vi "SPI API - SPI Simulation.vi"() -> ()   [LabVIEW 2014]
uses:
  Controls/Digital Data.ctl
  Controls/Timing Characteristics.ctl
panel:
  in  "SPI PHY Settings":T1={"Divide Value"=10, "Transfer Length (bits)"=24, "CS Asserted Polarity"=FALSE, "Clock Polarity (CPOL)"=FALSE, "Clock Phase (CPHA)"=FALSE, "Lengthen MISO Setup"=FALSE, "Direction Change Bit"=0, "MOSI Starts as Output"=FALSE, "Tristatable MOSI"=FALSE}
  in  "Chip Select":u8
  in  "Engine Rate (MHz)":i32=120
  out "Data To Slave":u64 format="%b"
  out "Timing Characteristics":T2 {"tCL (ns)" format="%#_4g"; "tCH (ns)" format="%#_4g"; "tCSS (ns)" format="%#_4g"; "tCSH (ns)" format="%#_4g"; "tCSW (ns)" format="%#_4g"; "Actual Sample Rate (Hz)" format="%_4p"; "SCLK Frequency (Hz)" format="%#.2p"}
  in  "Pause":bool
  in  "Sample Rate (Hz)":u32=100000 format="%.0p"
  out "Digital Data":digitalwaveform(graph)
  in  "Data To Slave":u64 format="%x"
  in  "Stop":bool
  # "Operating Instructions\n1. For this VI to work, the FPGA must be in Simulation Mode.\n2. Set the 'Engine Rate' control value to match your FPGA SPI Engine loop rate.\n3. Select a sample rate to control how often the SPI message is transmitted.\n4. Run the VI and observe the Timing Characterstics to the right."
  # "Typical Timing Diagram"
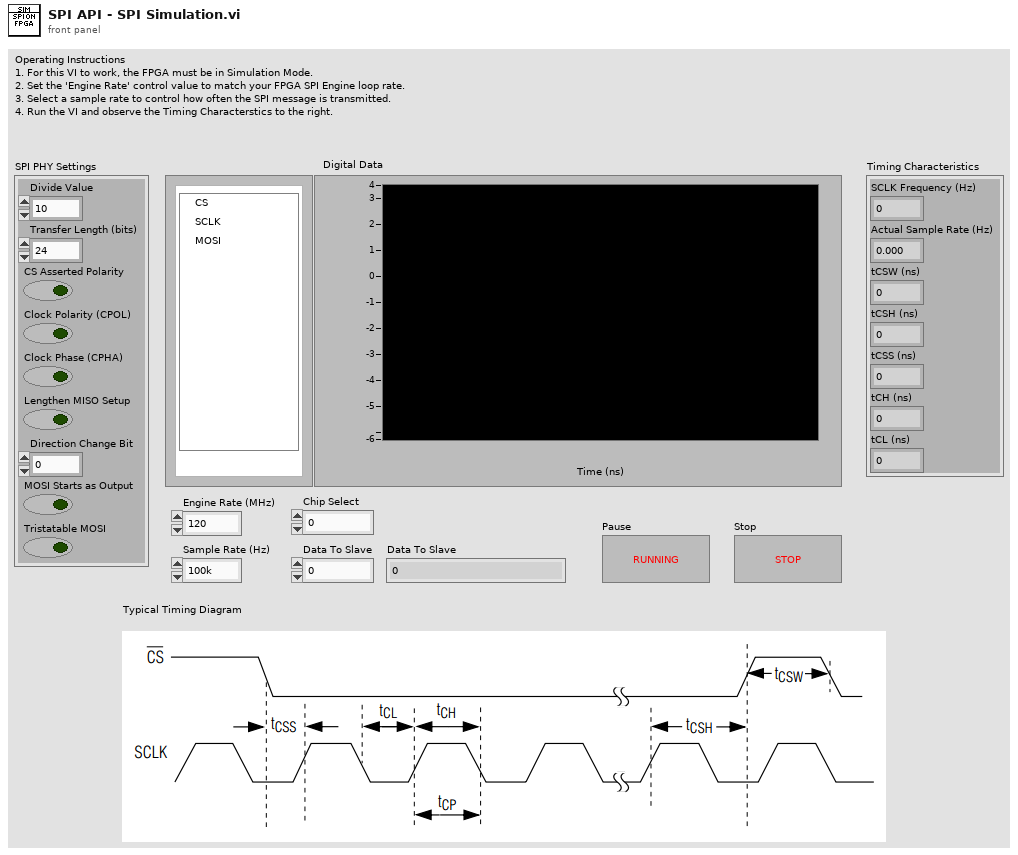
[diagram p1: front panel]
types:
  T1 = cluster{"Divide Value":u8, "Transfer Length (bits)":u8, "CS Asserted Polarity":bool, "Clock Polarity (CPOL)":bool, "Clock Phase (CPHA)":bool, "Lengthen MISO Setup":bool, "Direction Change Bit":u8, "MOSI Starts as Output":bool, "Tristatable MOSI":bool}
  T2 = typedef "Timing Characteristics.ctl" = cluster{"SCLK Frequency (Hz)":dbl, "Actual Sample Rate (Hz)":dbl, "tCSW (ns)":dbl, "tCSH (ns)":dbl, "tCSS (ns)":dbl, "tCH (ns)":dbl, "tCL (ns)":dbl}
  T3 = typedef "Digital Data.ctl" = cluster{"CS":bool, "SCLK":bool, "MISO":bool}
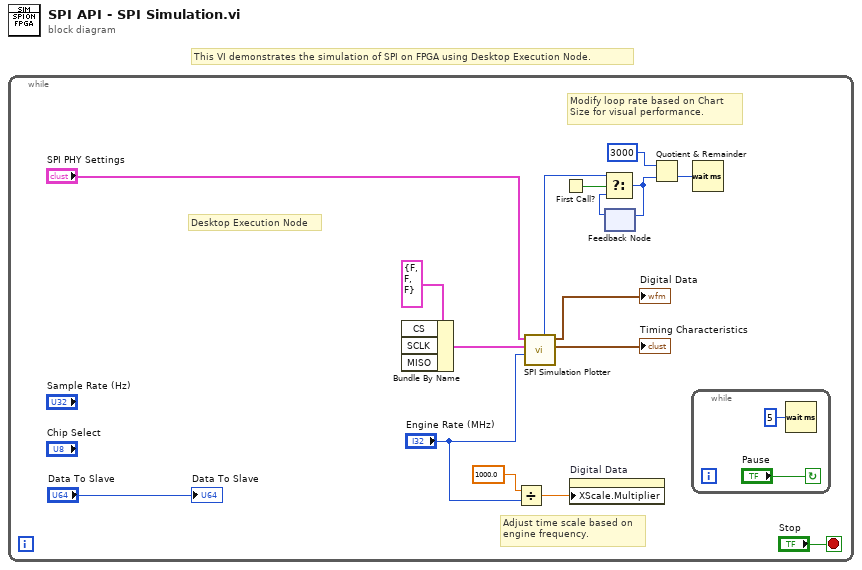
[diagram p0: block diagram]
diagram:
  # "This VI demonstrates the simulation of SPI on FPGA using Desktop Execution Node."
  n1 = while {
    stop <- "Stop" stop-if-true
    # "Adjust time scale based on\nengine frequency."
    # "Desktop Execution Node"
    # "Modify loop rate based on Chart\nSize for visual performance."
    n2 = Bundle By Name(cluster=T3 {"CS"=FALSE, "SCLK"=FALSE, "MISO"=FALSE}) -> (w9:T3)  [unwired: 3 in]
    n3 = Divide(x=1000.0, y="Engine Rate (MHz)") -> (x/y=w3:dbl)
    n4 = call "SPI Simulation Plotter.vi"("Engine Clock Rate (MHz)"="Engine Rate (MHz)", "SPI Signals"=w9, "SPI PHY Settings"="SPI PHY Settings") -> ("Timing Characteristics"=→"Timing Characteristics":T2, "Digital Data"=→"Digital Data":digitalwaveform, "Chart Size"=w8:i32)  [unwired: 6 in]
    n5 = First Call?() -> (First Call?: T/F=w14:bool)
    n6 = property on="Digital Data" class="DigitalGraph (strict)"("XScale.Multiplier"=w3) -> ()  [unwired: 2 in, 2 out]
    n7 = feedback #1() -> (w13:i32)  [unwired: 1 in]
    n8 = Select(t=w8, s=w14, f=w13) -> (s? t:f=w12:i32)
    n9 = feedback-in #1(w12) -> ()
    n10 = Quotient & Remainder(x=u32 3000 ("ms per Command"), y=w12) -> (floor(x/y)=w10:u32)  [unwired: 1 out]
    n11 = while {
      stop <- "Pause" continue-if-true
      n12 = Wait (ms)(milliseconds to wait=u32 5) -> ()  [unwired: 1 out]
    }
    n13 = Wait (ms)(milliseconds to wait=w10) -> ()  [unwired: 1 out]
    "Data To Slave" <- "Data To Slave"
  }
